vi "Convert Node Result to Test Suite - Assertion without Time - Time is relative to Registration Timestamp.vi"() -> ()   [LabVIEW 2013, in "JUnit Conversion Tests.lvlib"]
uses:
  JUnit Conversion Tests.lvlib
  <vilib>/addons/_JKI Toolkits/Caraya/classes/Assert/Assert.lvclass
  <vilib>/addons/_JKI Toolkits/Caraya/classes/Assert/Assert Equal Value_Variant.vi
  <vilib>/addons/_JKI Toolkits/Caraya/classes/Test/Test.lvclass
  JUnit Conversion/JUnit Conversion.lvlib
  <vilib>/addons/_JKI Toolkits/Caraya/classes/Test Result/Test Registration Data.ctl
  <vilib>/addons/_JKI Toolkits/Caraya/classes/Test Result/Test Result.lvclass
  <vilib>/addons/_JKI Toolkits/Caraya/classes/Test Result/Test Node (Extended).ctl
  <vilib>/addons/_JKI Toolkits/Caraya/classes/Test Result/Assert Event Data (Extended).ctl
  <vilib>/addons/_JKI Toolkits/Caraya/classes/Test Result/Node Results (Extended).ctl
  <vilib>/addons/_JKI Toolkits/Caraya/classes/MsgSerializer/MsgSerializer.lvclass
  <vilib>/PNR/JUnit XML/JUnit XML/Test Suite/Test Suite.lvclass
  <vilib>/PNR/JUnit XML/JUnit XML/Test Case/Test Case.lvclass
panel:
  out "error out":errorcluster
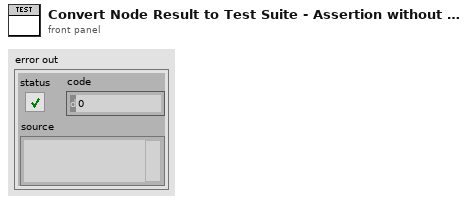
[diagram p1: front panel]
types:
  T1 = typedef "Caraya.lvlib/Test Result.lvclass/Assert Event Data (Extended).ctl" = cluster{"name":string, "passed":bool, "call-chain":string[], "test-error":errorcluster, "timestamp":timestamp, "assert-id":string, "test-id":string, "time":dbl, "message":string, "properties":variant, "measurements":variant, "user-defined":variant}
  T2 = typedef "Caraya.lvlib/Test Result.lvclass/Node Results (Extended).ctl" = cluster{"Test Node":T3, "Assertions":T1[]}
  T3 = typedef "Caraya.lvlib/Test Result.lvclass/Test Node (Extended).ctl" = cluster{"Test Registration":T4, "Defined":bool, "Passed":bool, "properties":variant}
  T4 = typedef "Caraya.lvlib/Test Result.lvclass/Test Registration Data.ctl" = cluster{"Name":string, "Call Chain":string[], "Time Stamp":timestamp, "Test ID":string, "Caller ID":string}
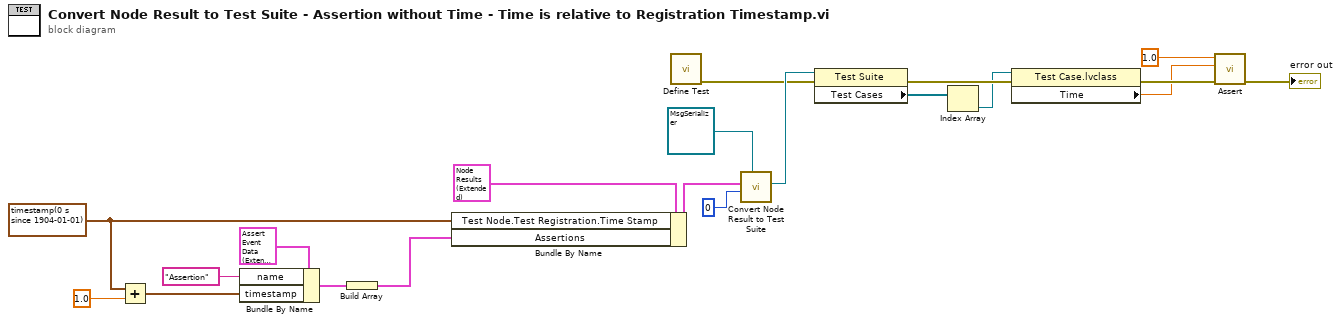
[diagram p0: block diagram]
diagram:
  w6 = timestamp(0 s since 1904-01-01) ("Test Node.Test Registration.Time Stamp")
  n1 = Add(x=w6, y=1.0) -> (x+y=w7:timestamp)
  n2 = Bundle By Name(cluster=T1 {"name"="", "passed"=FALSE, "call-chain"=[], "test-error"={"status"=FALSE, "code"=0, "source"=""}, "timestamp"=timestamp(0 s since 1904-01-01), "assert-id"="", "test-id"="", "time"=0.0, "message"="", "properties"=variant, "measurements"=variant, "user-defined"=variant} ("Assert Event Data"), "name"="Assertion", "timestamp"=w7) -> (w9:T1)
  n3 = Build Array(w9) -> (w8:T1[])
  n4 = Bundle By Name(cluster=T2 {"Test Node"={"Test Registration"={"Name"="", "Call Chain"=[], "Time Stamp"=timestamp(0 s since 1904-01-01), "Test ID"="", "Caller ID"=""}, "Defined"=FALSE, "Passed"=FALSE, "properties"=variant}, "Assertions"=[]} ("Node Result"), "Test Node.Test Registration.Time Stamp"=w6, "Assertions"=w8) -> (w13:T2)
  n5 = call <vilib>:"Define Test.vi"() -> ("error out"=w18:errorcluster)  [unwired: 10 in, 1 out]
  n6 = call "Convert Node Result to Test Suite.vi"("MsgSerializer"=refnum<class "MsgSerializer.lvclass"> refnum, "ID"=0, "Node Result"=w13) -> ("Test Suite"=w20:refnum<class "Test Suite.lvclass">)  [unwired: 8 in]
  n7 = property class="Test Suite"(reference=w20, error in=w18) -> (error out=w19:errorcluster, "Test Cases"=w3:refnum<class "Test Case.lvclass">[])  [unwired: 1 out]
  n8 = Index Array(array=w3) -> (element=w2:refnum<class "Test Case.lvclass">)  [unwired: 1 in]
  n9 = property class="Test Case.lvclass"(reference=w2, error in=w19) -> (error out=w4:errorcluster, "Time"=w1:dbl)  [unwired: 1 out]
  n10 = call-poly <vilib>:"Assert.vi"("error in (no error)"=w4, "Actual"=w1, "Expected"=1.0 ("size(s)")) -> ("error out"=→"error out":errorcluster)  [unwired: 7 in, 1 out]
